vi "BUNDLE BY NAME AND UNBUNDLE BY NAME.vi"() -> ()   [LabVIEW 2019]
panel:
  in  "GENDER 2":bool
  in  "SALARY 2":u16
  in  "NAME 2":string
  out "output cluster":T1
  in  "Cluster 2":T1
  in  "AGE 2":u8
  out "GENDER":bool
  out "SALARY":u16
  out "AGE":u8
  out "NAME":string
  in  "Cluster":T1
  # "BUNDLE BY NAME AND  UNBUNDLE BY NAME"
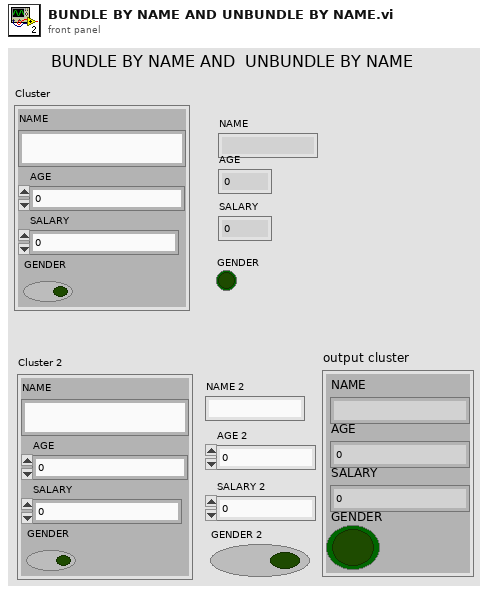
[diagram p1: front panel]
types:
  T1 = cluster{"NAME":string, "AGE":u8, "SALARY":u16, "GENDER":bool}
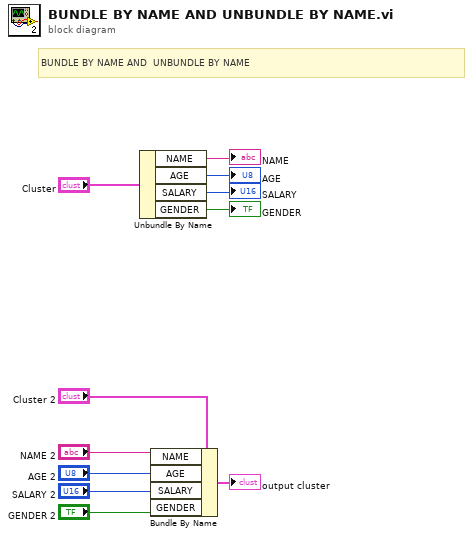
[diagram p0: block diagram]
diagram:
  # "BUNDLE BY NAME AND  UNBUNDLE BY NAME"
  n1 = Unbundle By Name("Cluster") -> ("NAME"=→"NAME":string, "AGE"=→"AGE":u8, "SALARY"=→"SALARY":u16, "GENDER"=→"GENDER":bool)
  n2 = Bundle By Name(cluster="Cluster 2", "NAME"="NAME 2", "AGE"="AGE 2", "SALARY"="SALARY 2", "GENDER"="GENDER 2") -> (→"output cluster":T1)
